vi "Boiler System Open.vi"(8 "error in":errorcluster) -> (0 "error out":errorcluster)   [LabVIEW 2015]
uses:
  Exercise 3-2/Course Project/support/User Event - Stop/User Event - Stop.lvlib
  Exercise 3-2/Course Project/support/Message Queue/Message Queue.lvlib
panel:
  out "String 3":string
  out "String 2":string
  out "String":string
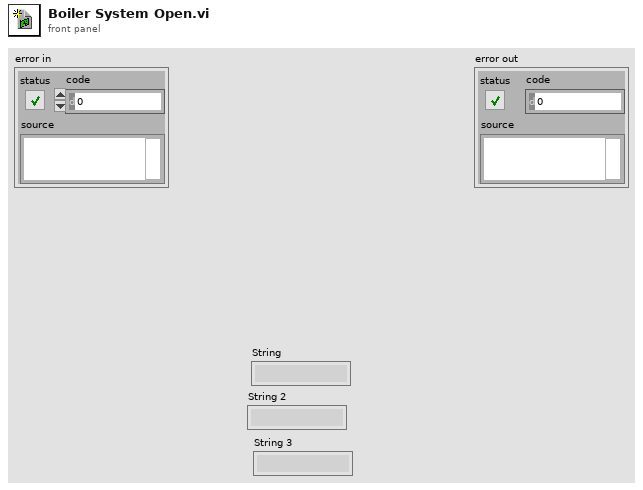
[diagram p1: front panel]
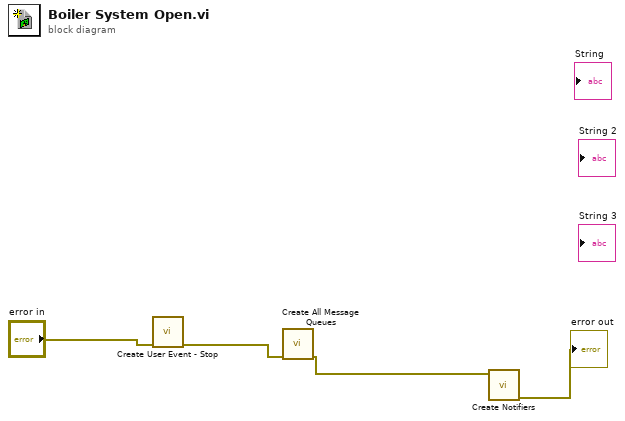
[diagram p0: block diagram]
diagram:
  n1 = call "Create User Event - Stop.vi"("error in (no error)"="error in") -> ("error out"=w3:errorcluster)  [unwired: 8 in, 2 out]
  n2 = call "Create All Message Queues.vi"("error in"=w3) -> ("error out"=w2:errorcluster)  [unwired: 9 in, 1 out]
  n3 = call "Create Notifiers.vi"("error in"=w2) -> ("error in 2"=→"error out":errorcluster)  [unwired: 10 in]
